vi "Read Binary File.vi"() -> ()   [LabVIEW 2023]
doc: "Reads an array of data from a byte stream binary file. By default, the VI is configured to read 8-byte (data type DBL) Little Endian Data. To modify the way sample data is read from the file, change the Byte Order and the value of the Byte Size (normal sizes are 1, 2, 4, or 8). If you change the byte size, also change the representation of the Data Type constant (default is DBL) to coincide with the byte size (1 = I8, 2 = I16, 4 = I32, 8 = DBL). Use the Write Binary File VI to create the file."
panel:
  out "Data Read from File":dbl[](graph)
  # "Overview: Demonstrates the use of the File I/O functions to read data from a binary file.\nInstructions:\n1. Make sure you have already run Write Binary File.vi.\n2. Run this VI. The contents of the binary file will be displayed below.\n3. Delete the binary file (located at [LabVIEW Data]\\Example Binary File.dat) when you are done."
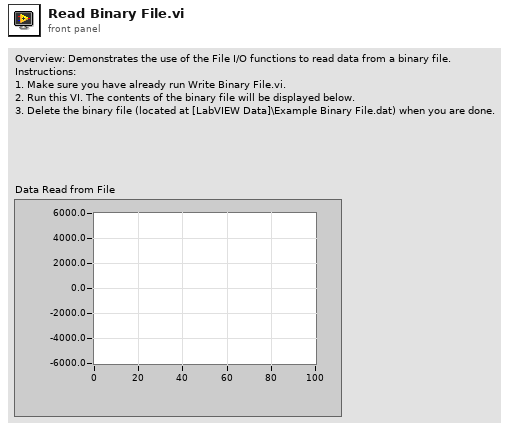
[diagram p1: front panel]
types:
  T1 = enum16{"open", "replace", "create", "open or create", "replace or create", "replace or create with confirmation"}
  T2 = enum16{"big-endian, network order", "native, host order", "little-endian"}
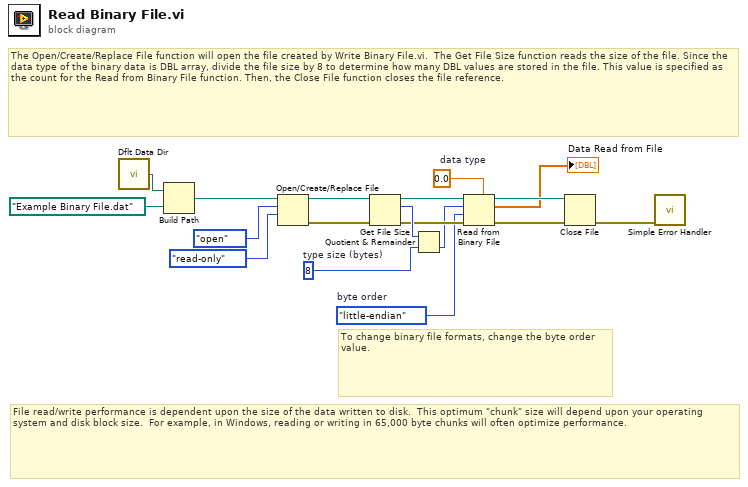
[diagram p0: block diagram]
diagram:
  w8 = T2."little-endian"  # byte order
  w10 = i64 8  # type size (bytes)
  w11 = 0.0  # data type
  # "File read/write performance is dependent upon the size of the data written to disk.  This optimum \"chunk\" size will depend upon your operating system and disk block size.  For example, in Windows, reading or writing in 65,000 byte chunks will often optimize performance."
  # "To change binary file formats, change the byte order value."
  # "The Open/Create/Replace File function will open the file created by Write Binary File.vi.  The Get File Size function reads the size of the file. Since the data type of the binary data is DBL array, divide the file size by 8 to determine how many DBL values are stored in the file. This value is specified as the count for the Read from Binary File function. Then, the Close File function closes the file reference."
  n1 = call <vilib>:"Dflt Data Dir.vi"() -> ("App:Default Data Directory"=w6:path)
  n2 = Build Path(base path=w6, name or relative path=path "Example Binary File.dat" ("default name")) -> (appended path=w4:path)
  n3 = Open/Create/Replace File(file path (use dialog)=w4, operation (0:open)=T1."open", access (0:read/write)=enum16{"read/write", "read-only", "write-only"}."read-only") -> (refnum out=w2:refnum<file>, error out=w3:errorcluster)  [unwired: 3 in, 1 out]
  n4 = Get File Size(file=w2, error in=w3) -> (refnum out=w18:refnum<file>, size (in bytes)=w15:i64, 0:w14:errorcluster)
  n5 = Quotient & Remainder(x=w15, y=w10) -> (floor(x/y)=w9:i64)  [unwired: 1 out]
  n6 = Read from Binary File(5:w11, 8:w14, 9:w8, 10:w9, 11:w18) -> (0:w16:errorcluster, 2:→"Data Read from File":dbl[], 3:w17:refnum<file>)  [unwired: 1 in, 1 out]
  n7 = Close File(refnum=w17, error in=w16) -> (error out=w1:errorcluster)  [unwired: 1 out]
  n8 = call <vilib>:"Simple Error Handler.vi"("error in (no error)"=w1) -> ()  [unwired: 4 in, 5 out]
